vi "Teardown Error Msg.vi"() -> (2 "Msg":refnum<class "Msg.lvclass">)   [LabVIEW 2020, in "jettl.lvlib" / "Teardown Error Msg.lvlib"]
uses:
  Teardown Error Msg.lvlib
  Msg/Msg.lvclass
  Teardown Error Msg/Teardown Error Msg.lvclass
  C:/git/jettl/src/jettl/jettl/Msg/Msg.lvclass
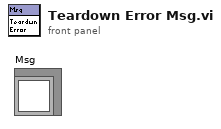
[diagram p1: front panel]
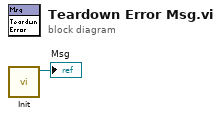
[diagram p0: block diagram]
diagram:
  n1 = call "Init.vi"() -> ("Teardown Error Msg out"=→"Msg":refnum<class "Teardown Error Msg.lvclass">)  [unwired: 11 in]
